vi "EncoderForwardNoPID.vi"(6 "Right axis value":dbl=-0.75 format="%#_13g", 8 "EncoderDevRef 4":T1={"DevStatus"={"status"=FALSE, "code"=0, "source"=""}, "EncoderIndex"=enum."Invalid", "CounterIndex"=enum."Ctr 1", "DistancePerCount"=2.0, "Decoding Type"=enum."4x"}, 9 "RobotDriveDevRef":T5={"DevStatus"={"status"=FALSE, "code"=0, "source"=""}, "Motors[]"=[], "Square Inputs"=FALSE, "Max Output"=1.0, "Isochronous"=FALSE}, 10 "EncoderDevRef":T1={"DevStatus"={"status"=FALSE, "code"=0, "source"=""}, "EncoderIndex"=enum."Invalid", "CounterIndex"=enum."Ctr 1", "DistancePerCount"=2.0, "Decoding Type"=enum."4x"}, 11 "Target":dbl format="%#_13g") -> (0 "EncoderDevRef 3":T1={"DevStatus"={"status"=FALSE, "code"=0, "source"=""}, "EncoderIndex"=enum."Invalid", "CounterIndex"=enum."Ctr 1", "DistancePerCount"=2.0, "Decoding Type"=enum."4x"}, 1 "RobotDriveDevRef 2":T5={"DevStatus"={"status"=FALSE, "code"=0, "source"=""}, "Motors[]"=[], "Square Inputs"=FALSE, "Max Output"=1.0, "Isochronous"=FALSE}, 2 "EncoderDevRef 2":T1={"DevStatus"={"status"=FALSE, "code"=0, "source"=""}, "EncoderIndex"=enum."Invalid", "CounterIndex"=enum."Ctr 1", "DistancePerCount"=2.0, "Decoding Type"=enum."4x"})   [LabVIEW 2013]
uses:
  <vilib>/Rock Robotics/WPI/RobotDrive/WPI_RobotDriveDevRef.ctl
  <vilib>/Rock Robotics/WPI/MotorControl/WPI_MotorControlDeviceRef.ctl
  <vilib>/Rock Robotics/SystemInterfaces/Typedef/FPGA_TypedefDigitalModule.ctl
  <vilib>/Rock Robotics/SystemInterfaces/DIO/FPGA_DIOPWMChannel.ctl
  <vilib>/Rock Robotics/WPI/PWM/WPI_PWMDeadband.ctl
  <vilib>/Rock Robotics/WPI/CAN/Jaguar/SubVIs/WPI_CANJaguar_ControlMode.ctl
  <vilib>/Rock Robotics/WPI/PWM/WPI_PWMTransform_ConPane.ctl
  <vilib>/Rock Robotics/WPI/Encoder/WPI_EncoderDevRef.ctl
  <vilib>/Rock Robotics/SystemInterfaces/Encoder/FPGA_EncoderIdx.ctl
  <vilib>/Rock Robotics/SystemInterfaces/Counter/FPGA_CounterCtrSystemIndex.ctl
  <vilib>/Rock Robotics/WPI/Encoder/WPI_EncoderType.ctl
  <vilib>/Rock Robotics/WPI/CAN/Jaguar/SubVIs/WPI_CANJaguar_BrakeCoastMode.ctl
panel:
  # "Stop?"
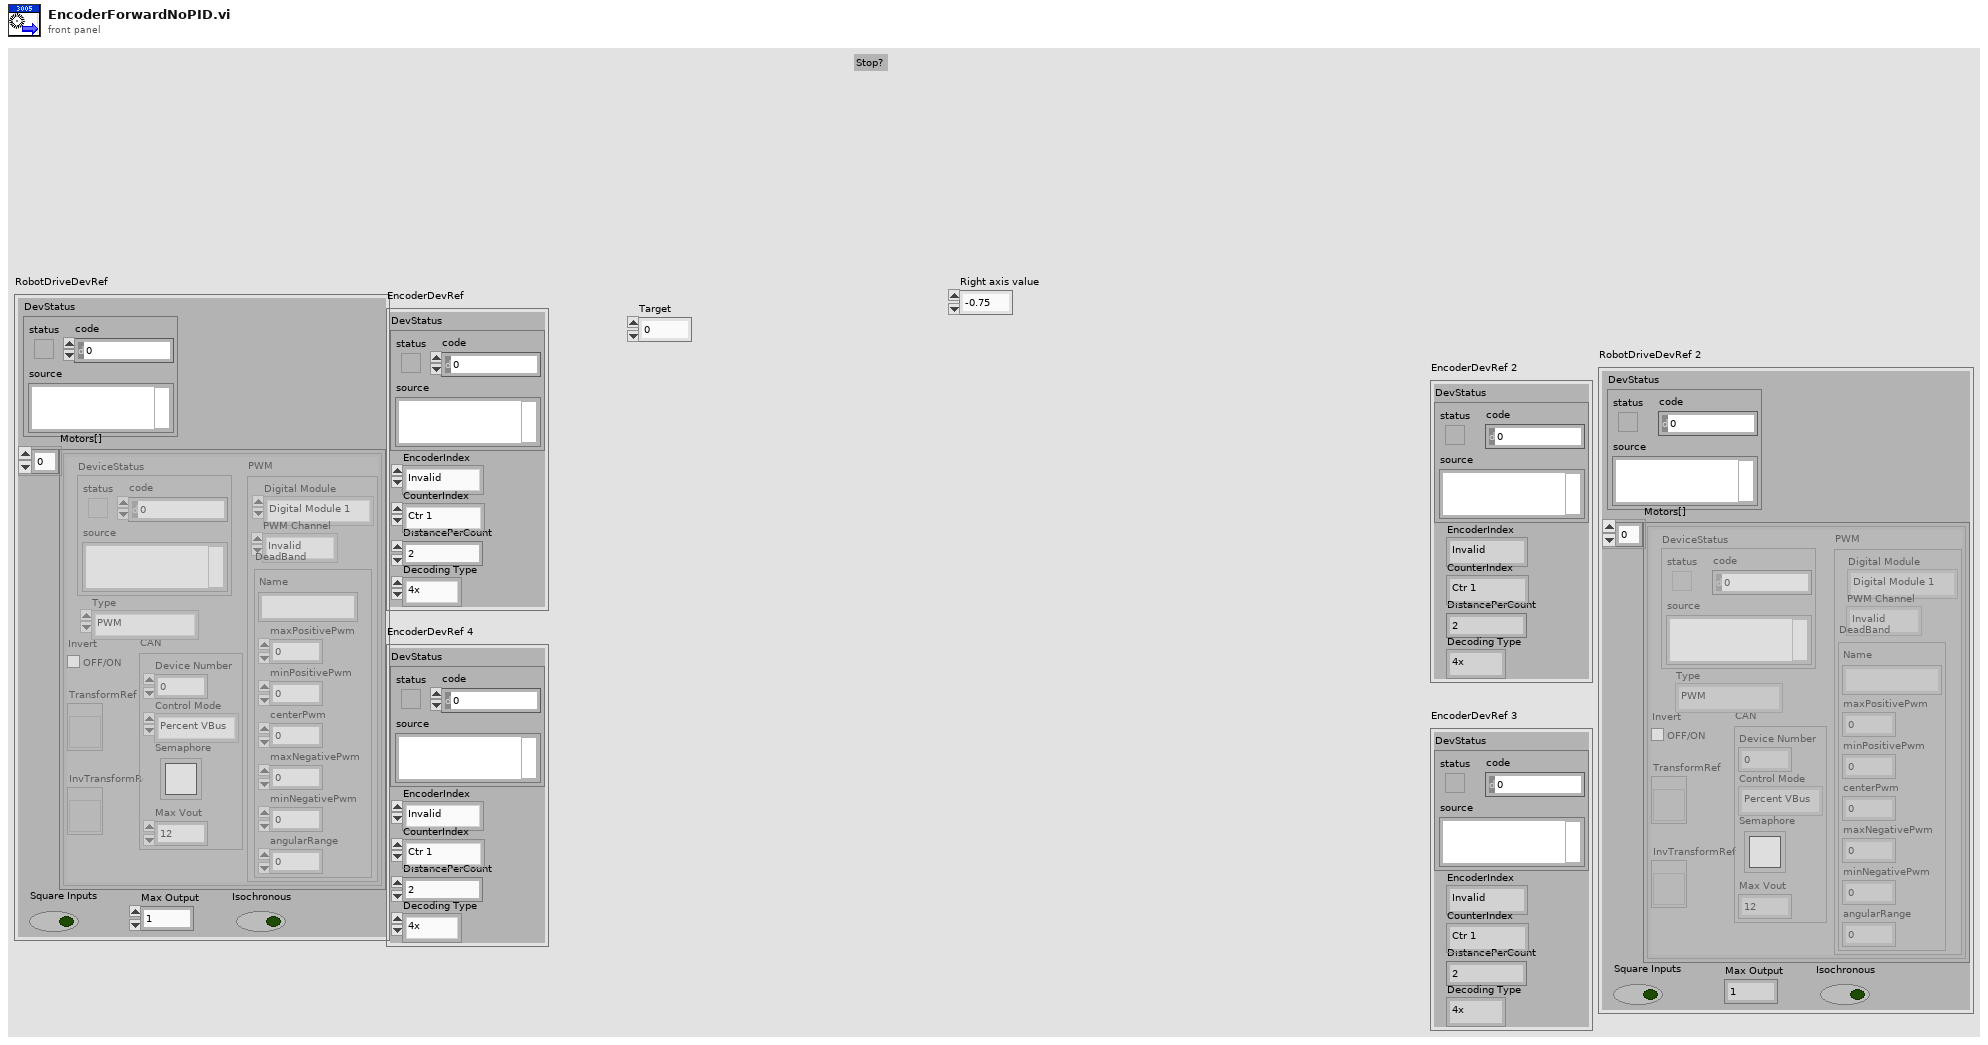
[diagram p1: front panel]
types:
  T1 = typedef "WPI_EncoderDevRef.ctl" = cluster{"DevStatus":errorcluster, "EncoderIndex":T2, "CounterIndex":T3, "DistancePerCount":dbl, "Decoding Type":T4}
  T2 = typedef "FPGA_EncoderIdx.ctl" = enum8{"Enc 0", "Enc 1", "Enc 2", "Enc 3", "Invalid"}
  T3 = typedef "FPGA_CounterCtrSystemIndex.ctl" = enum8{"Ctr 0", "Ctr 1", "Ctr 2", "Ctr 3", "Ctr 4", "Ctr 5", "Ctr 6", "Ctr 7", "Invalid"}
  T4 = typedef "WPI_EncoderType.ctl" = enum16{"1x", "2x", "4x"}
  T5 = typedef "WPI_RobotDriveDevRef.ctl" = cluster{"DevStatus":errorcluster, "Motors[]":T6[], "Square Inputs":bool, "Max Output":dbl, "Isochronous":bool}
  T6 = typedef "WPI_MotorControlDeviceRef.ctl" = cluster{"DeviceStatus":errorcluster, "Type":enum16{"PWM", "CAN"}, "PWM":cluster{"Digital Module":T7, "PWM Channel":T8, "DeadBand":T9}, "CAN":cluster{"Device Number":u8, "Control Mode":T10, "Semaphore":T11, "Max Vout":dbl}, "Invert":bool, "TransformRef":T12, "InvTransformRef":T12}
  T7 = typedef "FPGA_TypedefDigitalModule.ctl" = enum16{"Digital Module 1", "Digital Module 2"}
  T8 = typedef "FPGA_DIOPWMChannel.ctl" = enum8{"PWM 1", "PWM 2", "PWM 3", "PWM 4", "PWM 5", "PWM 6", "PWM 7", "PWM 8", "PWM 9", "PWM 10", "Invalid"}
  T9 = typedef "WPI_PWMDeadband.ctl" = cluster{"Name":string, "maxPositivePwm":i32, "minPositivePwm":i32, "centerPwm":i32, "maxNegativePwm":i32, "minNegativePwm":i32, "angularRange":u16}
  T10 = typedef "WPI_CANJaguar_ControlMode.ctl" = enum8{"Percent VBus", "Current", "Speed", "Position", "Voltage"}
  T11 = typedef "Semaphore RefNum" = refnum<k1>
  T12 = typedef "WPI_PWMTransform_ConPane.ctl" = refnum<vi>
  T13 = typedef "WPI_CANJaguar_BrakeCoastMode.ctl" = enum8{"Jumper", "Brake", "Coast"}
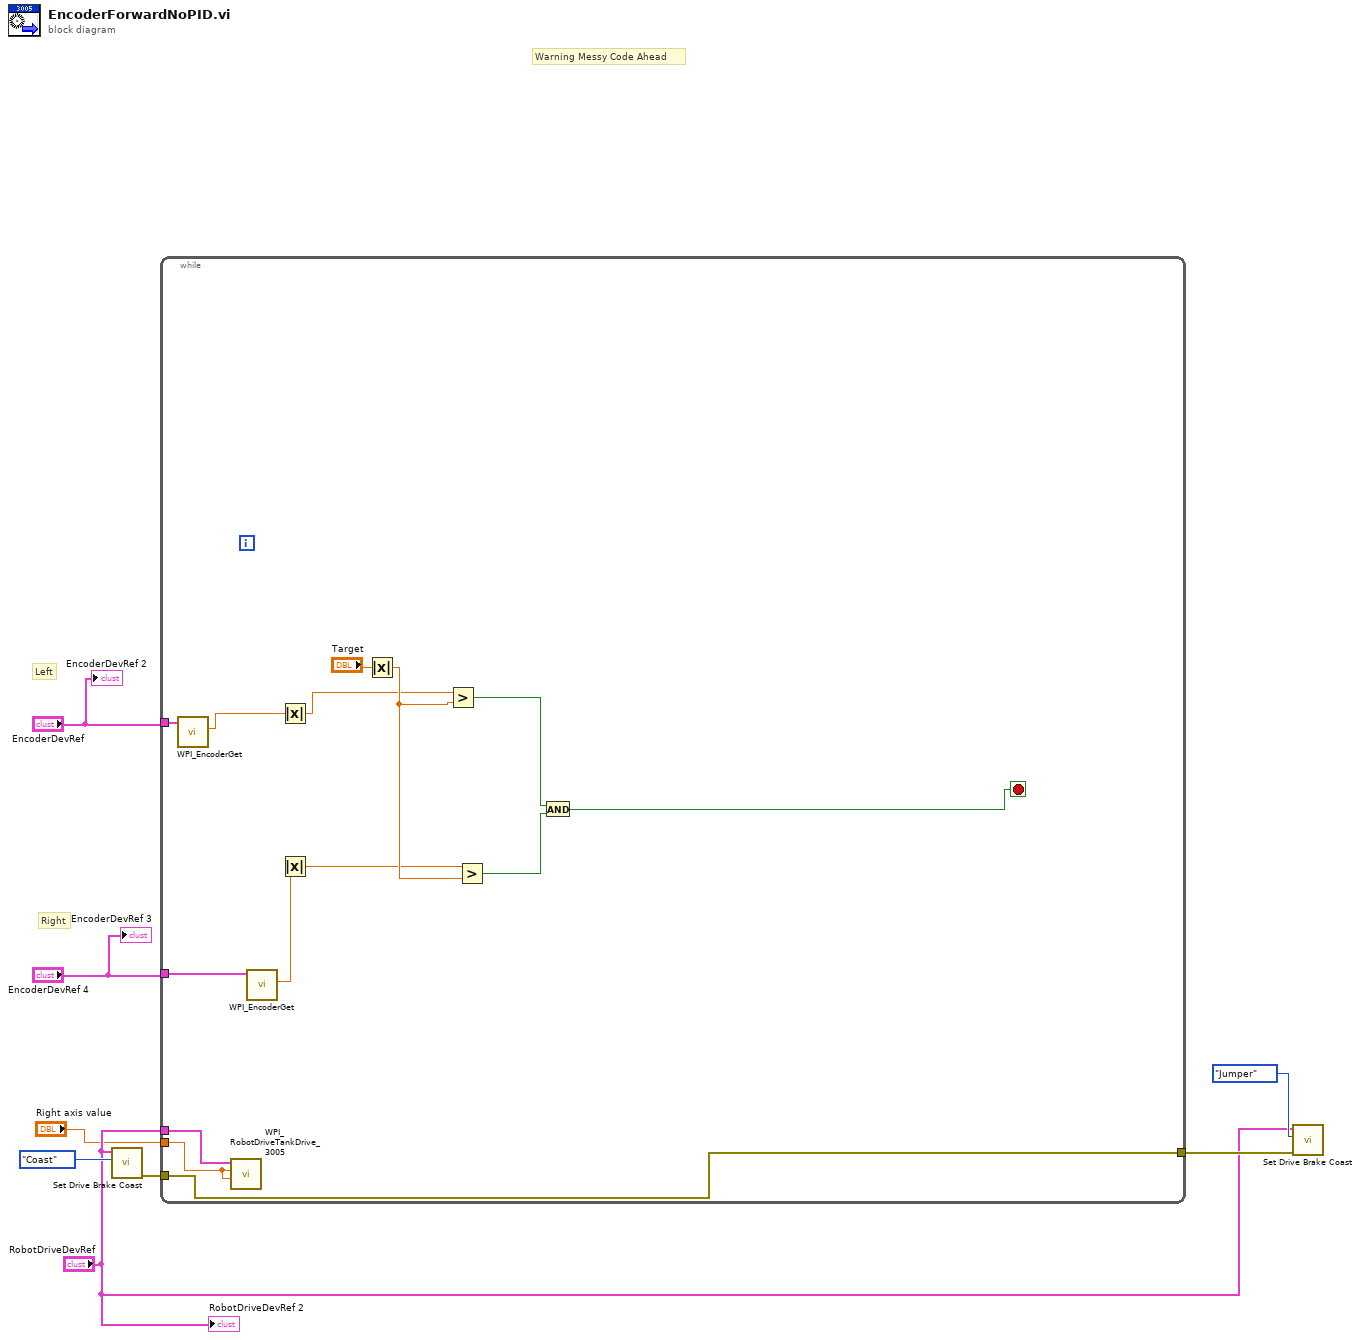
[diagram p0: block diagram]
diagram:
  # "Warning Messy Code Ahead"
  # "Right"
  # "Left"
  n1 = call "Set Drive Brake Coast.vi"("Brake / Coast Mode"=WPI_CANJaguar_BrakeCoastMode."Coast", "RobotDriveDevRef"="RobotDriveDevRef") -> ("error out"=w6:errorcluster)  [unwired: 8 in, 1 out]
  n2 = while {
    tunnel: "RobotDriveDevRef" -> [w22]
    tunnel: "EncoderDevRef" -> [w21]
    tunnel: "EncoderDevRef 4" -> [w20]
    tunnel: w6 -> [w10]
    tunnel: [w10] -> w4
    tunnel: "Right axis value" -> [w9]
    stop <- w17 stop-if-true
    n3 = call <vilib>:"WPI_EncoderGet.vi"("EncoderDevRef"=w21) -> ("Distance"=w14:dbl)  [unwired: 1 in, 9 out]
    n4 = call <vilib>:"WPI_RobotDriveTankDrive_3005.vi"("Right axis value"=w9, "Left axis value"=w9, "RobotDriveDevRef"=w22) -> ()  [unwired: 6 in, 3 out]
    n5 = call <vilib>:"WPI_EncoderGet.vi"("EncoderDevRef"=w20) -> ("Distance"=w12:dbl)  [unwired: 1 in, 9 out]
    n6 = Absolute Value(x=w14) -> (abs(x)=w13:dbl)
    n7 = Absolute Value(x=w12) -> (abs(x)=w11:dbl)
    n8 = Absolute Value(x="Target") -> (abs(x)=w15:dbl)
    n9 = Greater?(x=w13, y=w15) -> (0:w19:bool)
    n10 = Greater?(x=w11, y=w15) -> (0:w18:bool)
    n11 = And(x=w19, y=w18) -> (x .and. y?=w17:bool)
  }
  n12 = call "Set Drive Brake Coast.vi"("error in (no error)"=w4, "Brake / Coast Mode"=WPI_CANJaguar_BrakeCoastMode."Jumper", "RobotDriveDevRef"="RobotDriveDevRef") -> ()  [unwired: 7 in, 2 out]
  "RobotDriveDevRef 2" <- "RobotDriveDevRef"
  "EncoderDevRef 2" <- "EncoderDevRef"
  "EncoderDevRef 3" <- "EncoderDevRef 4"
